vi "setSettings.vi"(8 "error in (no error)":errorcluster, 10 "Settings":T1={"IP"="127.0.0.1", "port_low"=50000, "port_up"=50000, "connection_timeout "=10, "reading_timeout"=10, "writing_timeout"=10}, 11 "TCPSettings in":refnum<class "TCPSettings.lvclass">) -> (0 "error out":errorcluster, 3 "TCPSettings out":refnum<class "TCPSettings.lvclass">)   [LabVIEW 2016, in "TCPSettings.lvclass"]
uses:
  TCPSettings.lvclass
  tcpTypedefs/TCPSettings.ctl
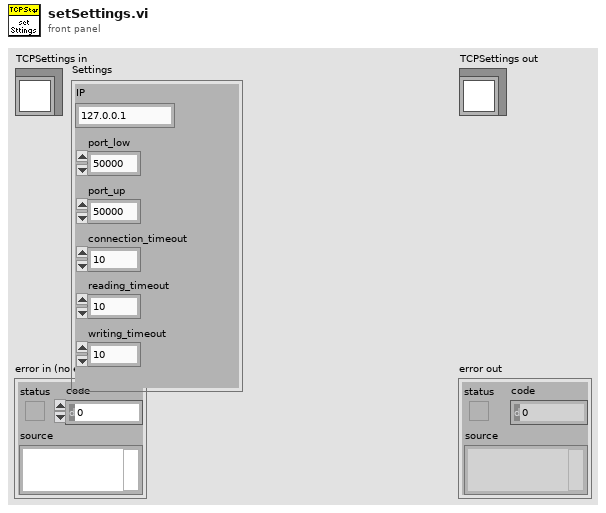
[diagram p1: front panel]
types:
  T1 = typedef "TCPSettings.ctl" = cluster{"IP":string, "port_low":u16, "port_up":u16, "connection_timeout ":i32, "reading_timeout":i32, "writing_timeout":i32}
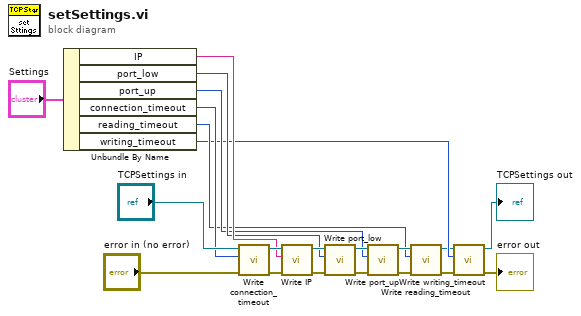
[diagram p0: block diagram]
diagram:
  n1 = Unbundle By Name("Settings") -> ("IP"=w7:string, "port_low"=w6:u16, "port_up"=w5:u16, "connection_timeout"=w8:i32, "reading_timeout"=w4:i32, "writing_timeout"=w3:i32)
  n2 = call-dynamic "Write connection_timeout .vi"("error in (no error)"="error in (no error)", "connection_timeout"=w8, "TCPSettings in"="TCPSettings in") -> ("error out"=w15:errorcluster, "TCPSettings out"=w12:refnum<class "TCPSettings.lvclass">)  [unwired: 7 in]
  n3 = call-dynamic "Write IP.vi"("error in (no error)"=w15, "IP"=w7, "TCPSettings in"=w12) -> ("error out"=w16:errorcluster, "TCPSettings out"=w11:refnum<class "TCPSettings.lvclass">)  [unwired: 7 in]
  n4 = call-dynamic "Write port_low.vi"("error in (no error)"=w16, "port_low"=w6, "TCPSettings in"=w11) -> ("error out"=w17:errorcluster, "TCPSettings out"=w10:refnum<class "TCPSettings.lvclass">)  [unwired: 7 in]
  n5 = call-dynamic "Write port_up.vi"("error in (no error)"=w17, "port_up"=w5, "TCPSettings in"=w10) -> ("error out"=w18:errorcluster, "TCPSettings out"=w9:refnum<class "TCPSettings.lvclass">)  [unwired: 7 in]
  n6 = call-dynamic "Write reading_timeout.vi"("error in (no error)"=w18, "reading_timeout"=w4, "TCPSettings in"=w9) -> ("error out"=w1:errorcluster, "TCPSettings out"=w2:refnum<class "TCPSettings.lvclass">)  [unwired: 7 in]
  n7 = call-dynamic "Write writing_timeout.vi"("error in (no error)"=w1, "writing_timeout"=w3, "TCPSettings in"=w2) -> ("error out"=→"error out":errorcluster, "TCPSettings out"=→"TCPSettings out":refnum<class "TCPSettings.lvclass">)  [unwired: 7 in]
